vi "FFT Measurement Test UI.vi"() -> ()   [LabVIEW 2014]
uses:
  <vilib>/rvi/interface/nirviMethod/nirviMethod.xnode
  <vilib>/FPGAPlugInAG/Dynamic/niLvFpga_ConfigureFifo_Dynamic.vi
  <vilib>/rvi/errors/niLvFpgaMergeErrorWithErrorCode.vi
  <vilib>/FPGAPlugInAG/Dynamic/niLvFpga_StartFifo_Dynamic.vi
  <vilib>/FPGAPlugInAG/Dynamic/niLvFpga_ReadFifo_Dynamic.vi
  <vilib>/rvi/Analysis/host/Public/NI_FpgaMspHost.lvlib
  <vilib>/rvi/interface/nirviOpenFPGA/nirviOpenFPGA.xnode
  <vilib>/rvi/interface/nirviCloseFPGA/nirviCloseFPGA.xnode
  <vilib>/FPGAPlugInAG/Dynamic/niLvFpga_Close_Dynamic.vi
  FPGA Target/Test VIs/FFT Measurement test.vi
panel:
  out "Gen. Freq.":dbl=10000000.0 format="%#_13g"
  in  "Sample Rate (S/s)":dbl=50000000.0 format="%#_13g"
  out "Error %":dbl
  out "Theoretical Freq.":dbl
  in  "#Periods":dbl=100.0
  in  "#Samples":dbl=1024.0
  out "Waveform Graph":dbl[](graph)
  out "Detected Frequency (Hz)":dbl
  out "Index Bin":dbl
  out "Signal":waveform(dbl)(graph)
  # "Theoretical Results"
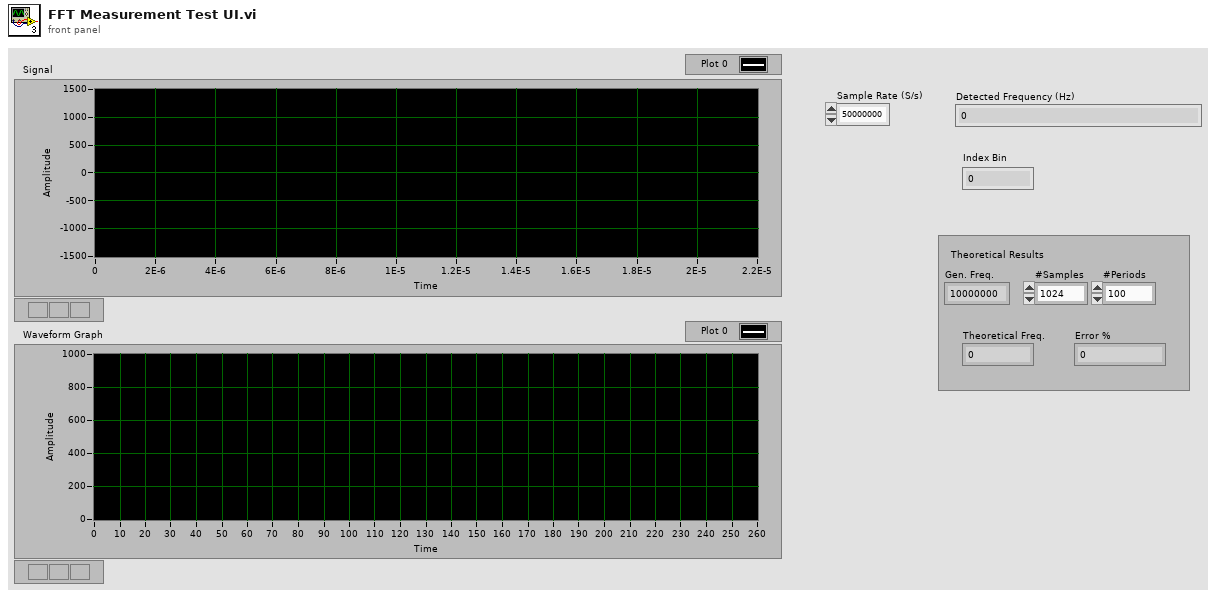
[diagram p1: front panel]
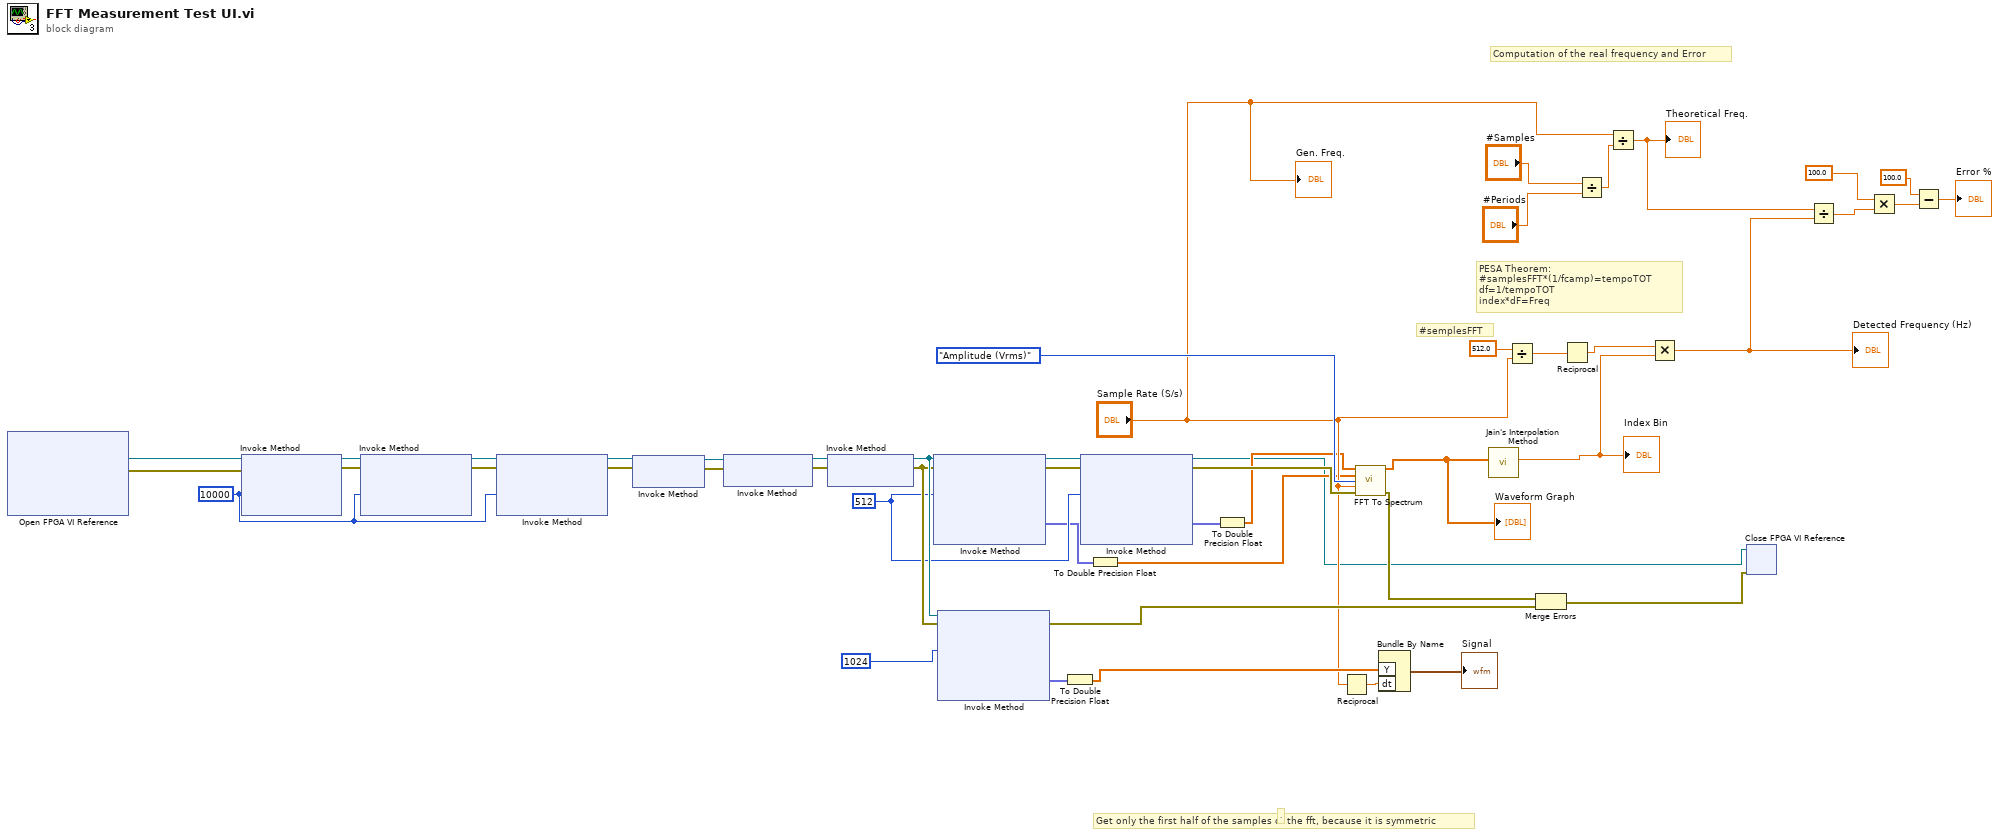
[diagram p0: block diagram]
diagram:
  w34 = u32 512 ("Requested Depth")
  w47 = u32 10000 ("Requested Depth")
  # "Computation of the real frequency and Error"
  # "."
  # "Get only the first half of the samples of the fft, because it is symmetric"
  # "#semplesFFT"
  # "PESA Theorem:\n#samplesFFT*(1/fcamp)=tempoTOT\ndf=1/tempoTOT\nindex*dF=Freq"
  n1 = xnode "Open FPGA VI Reference"() -> ("FPGA VI Reference Out"=w4:refnum<k20>, "error out"=w1:errorcluster)  [unwired: 2 in]
  n2 = xnode "Invoke Method"("FPGA VI Reference In"=w4, "error in"=w1, "Requested Depth"=w47) -> ("FPGA VI Reference Out"=w49:refnum<k20>, "error out"=w48:errorcluster)  [unwired: 1 out]
  n3 = xnode "Invoke Method"("FPGA VI Reference In"=w49, "error in"=w48, "Requested Depth"=w47) -> ("FPGA VI Reference Out"=w46:refnum<k20>, "error out"=w45:errorcluster)  [unwired: 1 out]
  n4 = xnode "Invoke Method"("FPGA VI Reference In"=w46, "error in"=w45, "Requested Depth"=w47) -> ("FPGA VI Reference Out"=w44:refnum<k20>, "error out"=w43:errorcluster)  [unwired: 1 out]
  n5 = xnode "Invoke Method"("FPGA VI Reference In"=w44, "error in"=w43) -> ("FPGA VI Reference Out"=w42:refnum<k20>, "error out"=w41:errorcluster)
  n6 = xnode "Invoke Method"("FPGA VI Reference In"=w42, "error in"=w41) -> ("FPGA VI Reference Out"=w37:refnum<k20>, "error out"=w40:errorcluster)
  n7 = xnode "Invoke Method"("FPGA VI Reference In"=w37, "error in"=w40) -> ("FPGA VI Reference Out"=w36:refnum<k20>, "error out"=w35:errorcluster)
  n8 = xnode "Invoke Method"("FPGA VI Reference In"=w36, "error in"=w35, "Number of Elements"=w34) -> ("FPGA VI Reference Out"=w39:refnum<k20>, "error out"=w38:errorcluster, "Data"=w26:fxp<+/-,22,22>[])  [unwired: 1 in, 1 out]
  n9 = xnode "Invoke Method"("FPGA VI Reference In"=w36, "error in"=w35, "Number of Elements"=u32 1024) -> ("error out"=w24:errorcluster, "Data"=w33:fxp<+/-,12,12>[])  [unwired: 1 in, 2 out]
  n10 = To Double Precision Float(number=w33) -> (double precision float=w31:dbl[])
  n11 = xnode "Invoke Method"("FPGA VI Reference In"=w39, "error in"=w38, "Number of Elements"=w34) -> ("FPGA VI Reference Out"=w3:refnum<k20>, "error out"=w29:errorcluster, "Data"=w27:fxp<+/-,22,22>[])  [unwired: 1 in, 1 out]
  n12 = To Double Precision Float(number=w26) -> (double precision float=w6:dbl[])
  n13 = To Double Precision Float(number=w27) -> (double precision float=w5:dbl[])
  n14 = Reciprocal(x="Sample Rate (S/s)") -> (1/x=w30:dbl)
  n15 = call <vilib>:"FFT To Spectrum.vi"("real FFT data"=w5, "imaginary FFT data"=w6, "spectrum type"=enum8{"Power (Vrms^2)", "Amplitude (Vrms)"}."Amplitude (Vrms)", "sample rate (S/s)"="Sample Rate (S/s)", "error in (no error)"=w29) -> ("spectrum out"=w19:dbl[], "error out"=w28:errorcluster)  [unwired: 8 in, 1 out]
  "Waveform Graph" <- w19
  n16 = Bundle By Name("Y"=w31, "dt"=w30) -> (→"Signal":waveform(dbl))  [unwired: 1 in]
  n17 = call "Jain's Interpolation Method.vi"("FFT array"=w19) -> ("Index Bin"=w21:dbl)  [unwired: 9 in, 1 out]
  "Index Bin" <- w21
  n18 = Divide(x=512.0, y="Sample Rate (S/s)") -> (x/y=w22:dbl)
  n19 = Merge Errors(w28, w24) -> (w2:errorcluster)
  n20 = Reciprocal(x=w22) -> (1/x=w20:dbl)
  n21 = Divide(x="#Samples", y="#Periods") -> (x/y=w18:dbl)
  n22 = Divide(x="Sample Rate (S/s)", y=w18) -> (x/y=w16:dbl)
  "Theoretical Freq." <- w16
  n23 = Multiply(x=w20, y=w21) -> (x*y=w17:dbl)
  "Detected Frequency (Hz)" <- w17
  n24 = xnode "Close FPGA VI Reference"("FPGA VI Reference In"=w3, "error in"=w2) -> ()  [unwired: 1 out]
  n25 = Divide(x=w16, y=w17) -> (x/y=w15:dbl)
  n26 = Multiply(x=100.0, y=w15) -> (x*y=w11:dbl)
  n27 = Subtract(x=100.0, y=w11) -> (x-y=→"Error %":dbl)
  "Gen. Freq." <- "Sample Rate (S/s)"
